vi "AlliGator Choose Harmonic Order Dialog.vi"(8 "error in (no error)":errorcluster) -> (0 "error out":errorcluster, 1 "OK":bool, 3 "Harmonic order":i32)   [LabVIEW 2021, in "AlliGator Phasor Graph.lvlib"]
doc: "Dialog to let the user enter the phasor frequency definition."
uses:
  AlliGator Phasor Graph.lvlib
panel:
  in  "Harmonic Order":i32=1 min=1 step=1
  out "String":string="Define phasor harmonic natural frequency order:"
  in  "OK":bool
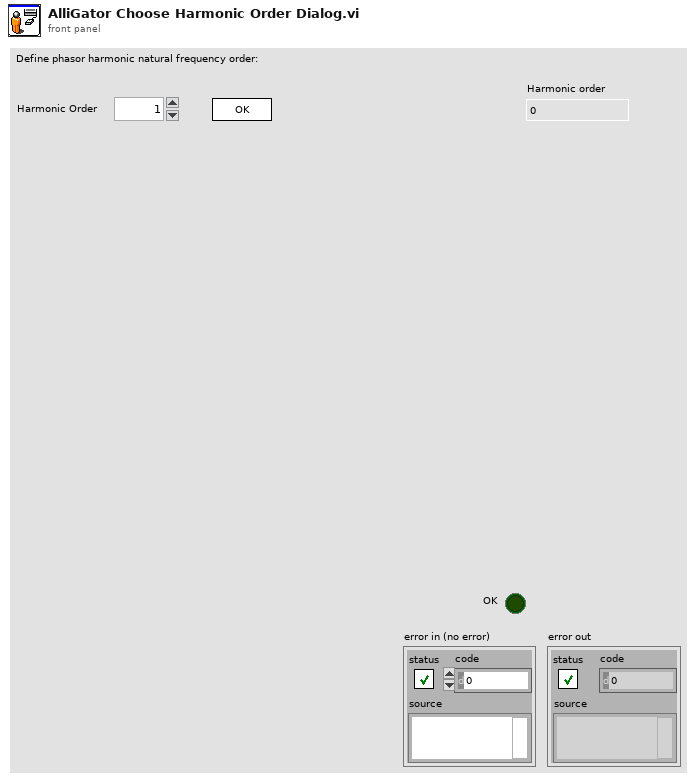
[diagram p1: front panel]
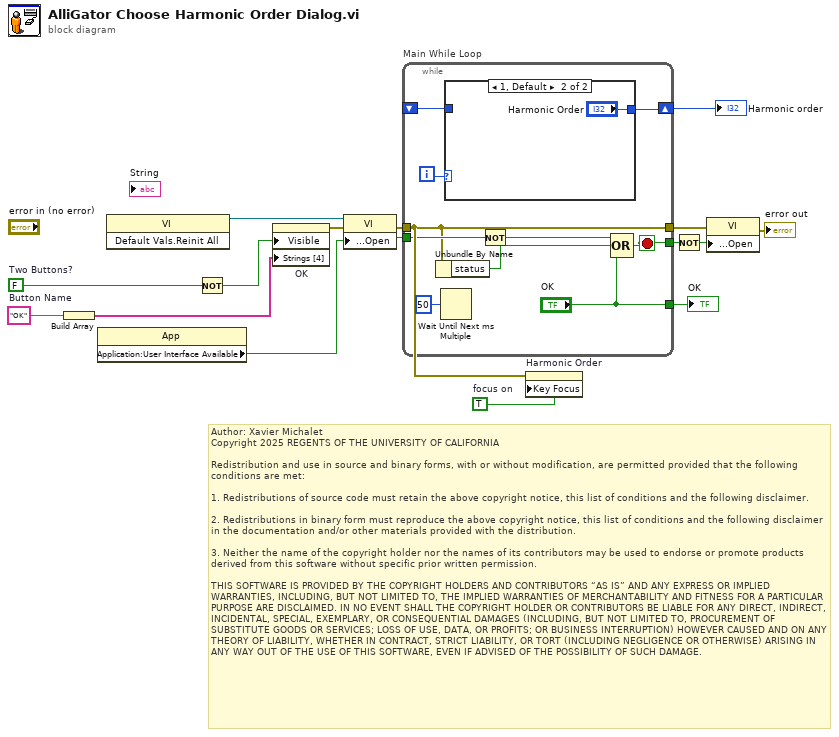
[diagram p0: block diagram]
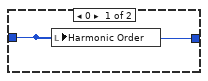
[diagram p2: hidden frame]
diagram:
  w2 = TRUE  # focus on
  w9 = "OK"  # Button Name
  w15 = FALSE  # Two Buttons?
  # "Author: Xavier Michalet\nCopyright 2025 REGENTS OF THE UNIVERSITY OF CALIFORNIA\n\nRedistribution and use in source and binary forms, with or without modification, are permitted provided that the following conditions are met:\n\n1. Redistributions of source code must retain the above copyright notice, this list of conditions and the following disclaimer.\n\n2. Redistributions in binary form must reproduce the above copyright notice, this list of conditions and the following disclaimer in the documentation and/or other materials provided with the distribution.\n\n3. Neither the name of the copyright holder nor the names of its contributors may be used to endorse or promote products derived from this software without specific prior written permission.\n\nTHIS SOFTWARE IS PROVIDED BY THE COPYRIGHT HOLDERS AND CONTRIBUTORS “AS IS” AND ANY EXPRESS OR IMPLIED WARRANTIES, INCLUDING, BUT NOT LIMITED TO, THE IMPLIED WARRANTIES OF MERCHANTABILITY AND FITNESS FOR A PARTICULAR PURPOSE ARE DISCLAIMED. IN NO EVENT SHALL THE COPYRIGHT HOLDER OR CONTRIBUTORS BE LIABLE FOR ANY DIRECT, INDIRECT, INCIDENTAL, SPECIAL, EXEMPLARY, OR CONSEQUENTIAL DAMAGES (INCLUDING, BUT NOT LIMITED TO, PROCUREMENT OF SUBSTITUTE GOODS OR SERVICES; LOSS OF USE, DATA, OR PROFITS; OR BUSINESS INTERRUPTION) HOWEVER CAUSED AND ON ANY THEORY OF LIABILITY, WHETHER IN CONTRACT, STRICT LIABILITY, OR TORT (INCLUDING NEGLIGENCE OR OTHERWISE) ARISING IN ANY WAY OUT OF THE USE OF THIS SOFTWARE, EVEN IF ADVISED OF THE POSSIBILITY OF SUCH DAMAGE."
  n1 = Build Array(w9) -> (w10:string[])
  n2 = property class="App"() -> ("Application:User Interface Available"=w4:bool)  [unwired: 2 in, 2 out]
  n3 = invoke class="VI" method="Default Vals.Reinit All"() -> (reference out=w3:refnum<vi>)  [unwired: 3 in, 2 out]
  n4 = Not(x=w15) -> (.not. x?=w13:bool)
  n5 = property on="OK" class="Bool"("Visible"=w13, "Strings [4]"=w10) -> (error out=w8:errorcluster)  [unwired: 2 in, 1 out]
  n6 = property class="VI"(reference=w3, error in=w8, "Front Panel Window:Open"=w4) -> (error out=w7:errorcluster)  [unwired: 1 out]
  n7 = while "Main While Loop" {
    tunnel: ["OK"] -> w14
    tunnel: w4 -> [w24]
    tunnel: [w22] -> w11
    tunnel: w7 -> [w21]
    tunnel: [w21] -> w6
    shift-right: [w18] -> w1
    shift-left: _ -> [w17]
    i -> [w19]
    stop <- w22 stop-if-true
    n8 = Unbundle By Name(w21) -> ("status"=w20:bool)
    n9 = Wait Until Next ms Multiple(millisecond multiple=u32 50) -> ()  [unwired: 1 out]
    n10 = case shown="1, Default" w19 {
      tunnel: [w26 "Harmonic Order"] -> w18
      tunnel: w17 -> [w26 _]
      frame 0 {
        n11 = local write "Harmonic Order"(w26) -> ()
      }
      frame 1, Default {
      }
    }
    n12 = Not(x=w24) -> (.not. x?=w23:bool)
    n13 = Compound Arithmetic op=OR(w23, w20, "OK") -> (w22:bool)
  }
  "OK" <- w14
  "Harmonic order" <- w1
  n14 = property on="Harmonic Order" class="DigNum (strict)"(error in=w7, "Key Focus"=w2) -> ()  [unwired: 1 in, 2 out]
  n15 = Not(x=w11) -> (.not. x?=w12:bool)
  n16 = property class="VI"(error in=w6, "Front Panel Window:Open"=w12) -> (error out=→"error out":errorcluster)  [unwired: 1 in, 1 out]
